vi "FGV_CtrlRef.vi"(8 "error in (no error)":errorcluster caption="entrée d'erreur (pas d'erreur)", 10 "CtrlsRefs_IN":T1[](array[typedef]), 11 "Action":T2=enum."GET") -> (0 "error out":errorcluster caption="sortie d'erreur", 2 "CtrlsRefs_OUT":T1[](array[typedef]))   [LabVIEW 2013]
uses:
  STANDARD/Action.ctl
  UTILS/CTL/CtrlRef.ctl
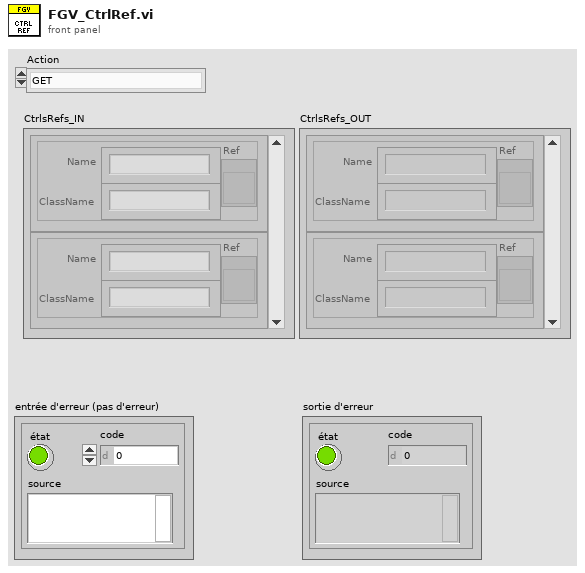
[diagram p1: front panel]
types:
  T1 = typedef "CtrlRef.ctl" = cluster{"Name":string, "Ref":refnum<vi>, "ClassName":string}
  T2 = typedef "Action.ctl" = enum16{"SET", "GET"}
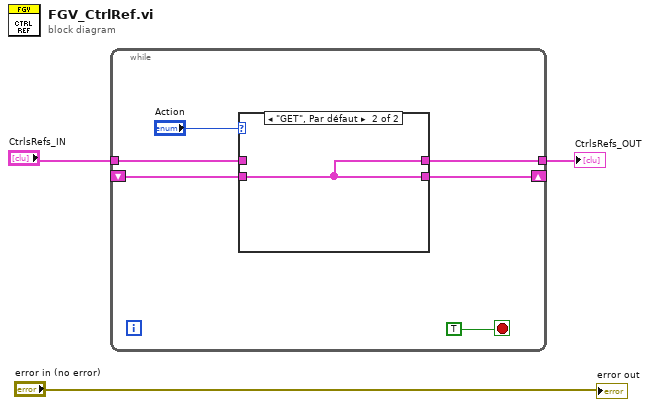
[diagram p0: block diagram]
diagram:
  n1 = while {
    shift-right: [w8] -> _
    shift-left: _ -> [w6]
    tunnel: "CtrlsRefs_IN" -> [w9]
    tunnel: [w7] -> w1
    stop <- TRUE stop-if-true
    n2 = case shown="\"GET\", Par défaut" "Action" {
      tunnel: w9 -> [w10 _]
      tunnel: [w10 w11] -> w8
      tunnel: [w10 w11] -> w7
      tunnel: w6 -> [_ w11]
      frame "SET" {
      }
      frame "GET", Default {
      }
    }
  }
  "CtrlsRefs_OUT" <- w1
  "error out" <- "error in (no error)"
